vi "Update_Waveform.vi"(0 "Data":T1={"ACQUIRED_DATA"={"Battery_Power"=0.0, "Power_Consumption"=0.0, "Inverter_Mode"=FALSE}, "Start"=TRUE, "Pause"=TRUE, "Record"=TRUE, "Low_Power"=TRUE, "Power_and_Power_Consumed"=[], "State_and_Data_In"={"State"="", "Data"=variant}, "File_Path"=path "", "Application_Directory"=path "", "Record_Select"=enum."Enabled", "Stop_Select"=enum."Enabled"}) -> (4 "Update_Data":T1={"ACQUIRED_DATA"={"Battery_Power"=0.0, "Power_Consumption"=0.0, "Inverter_Mode"=FALSE}, "Start"=TRUE, "Pause"=TRUE, "Record"=TRUE, "Low_Power"=TRUE, "Power_and_Power_Consumed"=[], "State_and_Data_In"={"State"="", "Data"=variant}, "File_Path"=path "", "Application_Directory"=path "", "Record_Select"=enum."Enabled", "Stop_Select"=enum."Enabled"})   [LabVIEW 2023]
doc: "Used to Update the Waveform with the Data"
uses:
  Controls/UPS_Data.ctl
  Controls/Acquired_Data.ctl
  Controls/State_and_Data.ctl
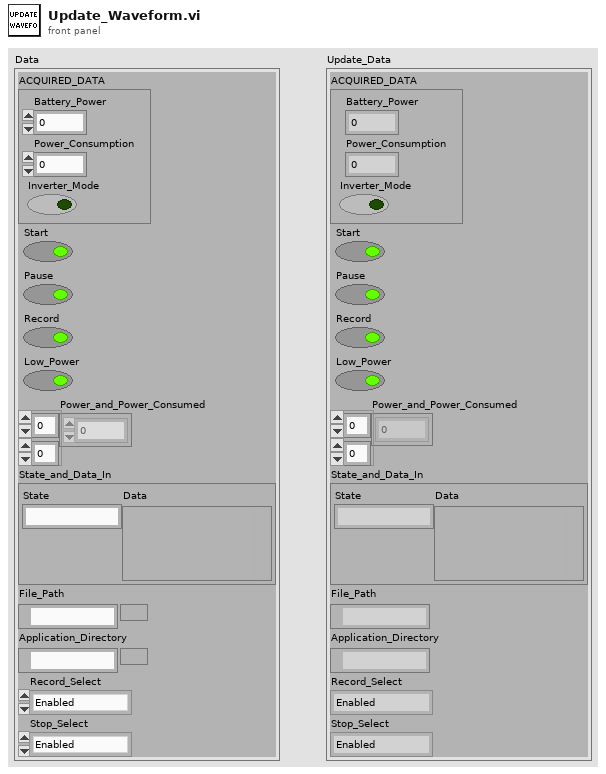
[diagram p1: front panel]
types:
  T1 = typedef "UPS_Data.ctl" = cluster{"ACQUIRED_DATA":T2, "Start":bool, "Pause":bool, "Record":bool, "Low_Power":bool, "Power_and_Power_Consumed":dbl[][], "State_and_Data_In":T3, "File_Path":path, "Application_Directory":path, "Record_Select":enum8{"Enabled", "Disabled", "Disabled and Grayed Out"}, "Stop_Select":enum8{"Enabled", "Disabled", "Disabled and Grayed Out"}}
  T2 = typedef "Acquired_Data.ctl" = cluster{"Battery_Power":dbl, "Power_Consumption":dbl, "Inverter_Mode":bool}
  T3 = typedef "State_and_Data.ctl" = cluster{"State":string, "Data":variant}
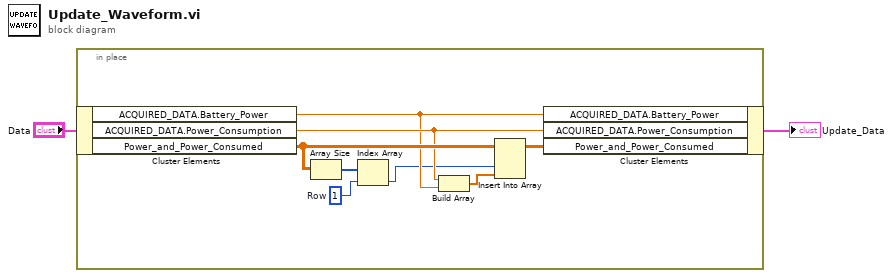
[diagram p0: block diagram]
diagram:
  n1 = in-place {
    w3 = 1  # Row
    n2 = in-place-cluster #1("Data") -> ("ACQUIRED_DATA.Battery_Power"=w6:dbl, "ACQUIRED_DATA.Power_Consumption"=w7:dbl, "Power_and_Power_Consumed"=w9:dbl[][])
    n3 = Array Size(array=w9) -> (size(s)=w8:i32[])
    n4 = Index Array(array=w8, index=w3) -> (element=w4:i32)
    n5 = Build Array(w7, w6) -> (w5:dbl[])
    n6 = Insert Into Array(array=w9, index (col)=w4, new element=w5) -> (w10:dbl[][])  [unwired: 1 in]
    n7 = in-place-cluster #1("ACQUIRED_DATA.Battery_Power"=w6, "ACQUIRED_DATA.Power_Consumption"=w7, "Power_and_Power_Consumed"=w10) -> (→"Update_Data":T1)
  }
